vi "Sample changer.vi"() -> ()   [LabVIEW 2016, in "Top Level.lvlib"]
uses:
  Top Level.lvlib
  Sample Changer 2008 BETA 3.10.3/Visual Readback/half extended piston (push).ctl
  Sample Changer 2008 BETA 3.10.3/Visual Readback/half extended piston (push-in).ctl
  Sample Changer 2008 BETA 3.10.3/Visual Readback/Sample Rod (mid).ctl
  Sample Changer 2008 BETA 3.10.3/Visual Readback/Sample Rod (up-cathode).ctl
  Sample Changer 2008 BETA 3.10.3/Visual Readback/Sample Rod (down).ctl
  Sample Changer 2008 BETA 3.10.3/Visual Readback/Wheel Gate Valve.ctl
  cRIO code/SCA/controls/Horizontal Rod states.ctl
  cRIO code/SCA/controls/Vertical Rod states.ctl
  controls/GV states.ctl
  cRIO code/SCA/controls/SCA broadcast status.ctl
  cRIO code/SCA/controls/SCA Bypass control.ctl
  cRIO code/SCA/controls/GP307 cluster.ctl
  cRIO code/SCA/controls/SCA commands.ctl
panel:
  in  "Tab Control":T1(tab)=enum."SCA Configuration"
  out "Sample Rod (down)":T2
  in  "Random Change":bool
  in  "Random rotate":bool
  in  "Open SC GV":bool
  in  "Close SC GV":bool
  in  "Raise sample rod":bool
  in  "Lower sample rod":bool
  in  "Retract retract rod":bool
  in  "Insert retract rod":bool
  in  "pump out system":bool
  in  "Retract insert rod":bool
  in  "Insert insert rod":bool
  in  "Requested sample":i16=1 min=1 max=64 step=1
  in  "rotate wheel":bool
  in  "change sample":bool
  in  "vent system":bool
  out "Extended Piston (out)":bool
  out "half extended piston (out)":T3
  out "Extended Piston (in)":bool
  out "half extended piston (in)":T4
  out "Sample Rod (mid)":T5
  out "Sample Rod (up)":T6
  out "Wheel Gate Valve":T7
  in  "stop":bool
  out "SCA Status":T8
  out "Status Message":string
  out "Wheel GV Status":T9
  out "Insert Rod Status":T10
  out "Retract Rod Status":T10
  out "Sample Rod status":T11
  out "Bellows Pressure":string
  out "Source Pressure":string
  out "Encoder position":i16
  out "New sample":i8
  out "Encoder Destination":i16
  out "Encoder position plot":i16(graph)
  in  "Time between data points (ms)":u32=100
  out "Encoder Position":u32
  out "Encoder Offset":i16
  out "Insert Rod Timeout":u32
  out "Retract Rod Timeout":u32
  out "Rollover Sample":i16
  out "Wheel GV Timeout":u32
  out "Step Window Radius":u8
  out "Rotate Wheel min Time":u32
  out "Sample Rod Timeout":u32
  out "Rotate Wheel timeout":u32
  in  "SM Config Update?":bool
  in  "Bypass Controls":T12
  out "Bypass Control Values":T12
  in  "Encoder Offset set":i16
  in  "Insert Rod Timeout set":u32
  in  "Retract Rod Timeout set":u32
  in  "Step Window Radius set":u8
  in  "Rollover Sample set":i16
  in  "Rotate Wheel min Time set":u32
  in  "Rotate Wheel timeout set":u32
  in  "Sample Rod Timeout set":u32
  in  "Wheel GV Timeout set":u32
  out "Shared Network Variable Error":errorcluster
  out "Change sample error":errorcluster
  out "SCA-RT error":errorcluster
  out "Rotate Wheel error":errorcluster
  out "SM command error":errorcluster
  out "Random change error":errorcluster
  out "Random rotate error":errorcluster
  out "SM Config Update error":errorcluster
  # "Opens or Closes Wheel chamber valve"
  # "rotate wheel or change sample"
  # "Inserts sample into wheel"
  # "Pushes sample out of wheel"
  # "Raises or lowers Sample Rod"
  # "vent system= isolate wheel chamber from bellows and source\nPump out system = re-connect wheel chamber to bellows and source"
  # "In order for new settings to take effect must press Update? button.\nAll time values are in ms.  Encoder items are in encoder steps (0-2^14)"
  # "If the cathode position is too low: You have to increase the value. Too high, you have to lower it.\n\nEncoder radius is the minimum number of steps allowed between desired and actual position\n\nRollover sample is defined as the last sample before the standard encoder conversion exceeds 2^14"
  # "Current Values"
  # "New Values"
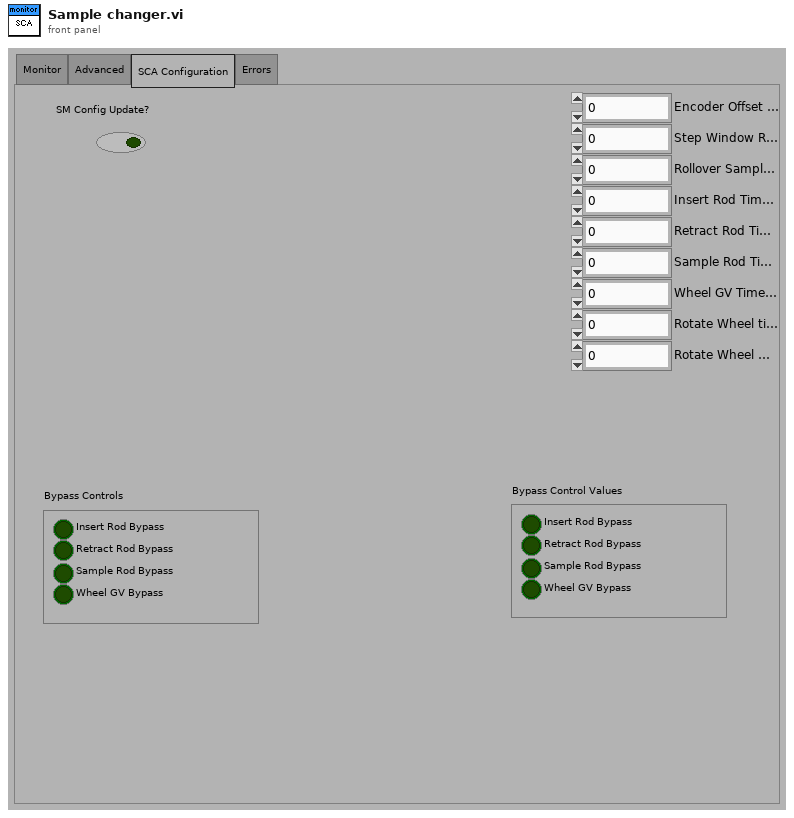
[diagram p1: front panel]
types:
  T1 = enum32{"Monitor", "Advanced", "SCA Configuration", "Errors"}
  T2 = typedef "Sample Rod (down).ctl" = bool
  T3 = typedef "half extended piston (push).ctl" = bool
  T4 = typedef "half extended piston (push-in).ctl" = bool
  T5 = typedef "Sample Rod (mid).ctl" = bool
  T6 = typedef "Sample Rod (up-cathode).ctl" = bool
  T7 = typedef "Wheel Gate Valve.ctl" = bool
  T8 = typedef "SCA broadcast status.ctl" = enum16{"Waiting", "Changing samples", "Sample change complete", "Failure"}
  T9 = typedef "GV states.ctl" = enum16{"status unclear", "closed", "open"}
  T10 = typedef "Horizontal Rod states.ctl" = enum16{"status unclear", "rod in", "rod out"}
  T11 = typedef "Vertical Rod states.ctl" = enum16{"status unclear", "rod down", "rod up"}
  T12 = typedef "SCA Bypass control.ctl" = cluster{"Insert Rod Bypass":bool, "Retract Rod Bypass":bool, "Sample Rod Bypass":bool, "Wheel GV Bypass":bool}
  T13 = typedef "SCA commands.ctl" = enum16{"Wait", "Shutdown", "Retract insert rod", "Insert insert rod", "Retract retract rod", "Insert retract rod", "Retract sample rod", "Insert sample rod", "Open wheel GV", "Close wheel GV", "Open ion source GV", "Close ion source GV", "Pump out source", "Vent source", "Rotate wheel randomly", "Rotate wheel", "Start random sample change", "Start sample change"}
  T14 = typedef "GP307 cluster.ctl" = cluster{"Ion gauge 1":string, "Convectron  Gauge 1 ":string, "Ion Gauge 2":string, "Convectrom Gauge 2":string}
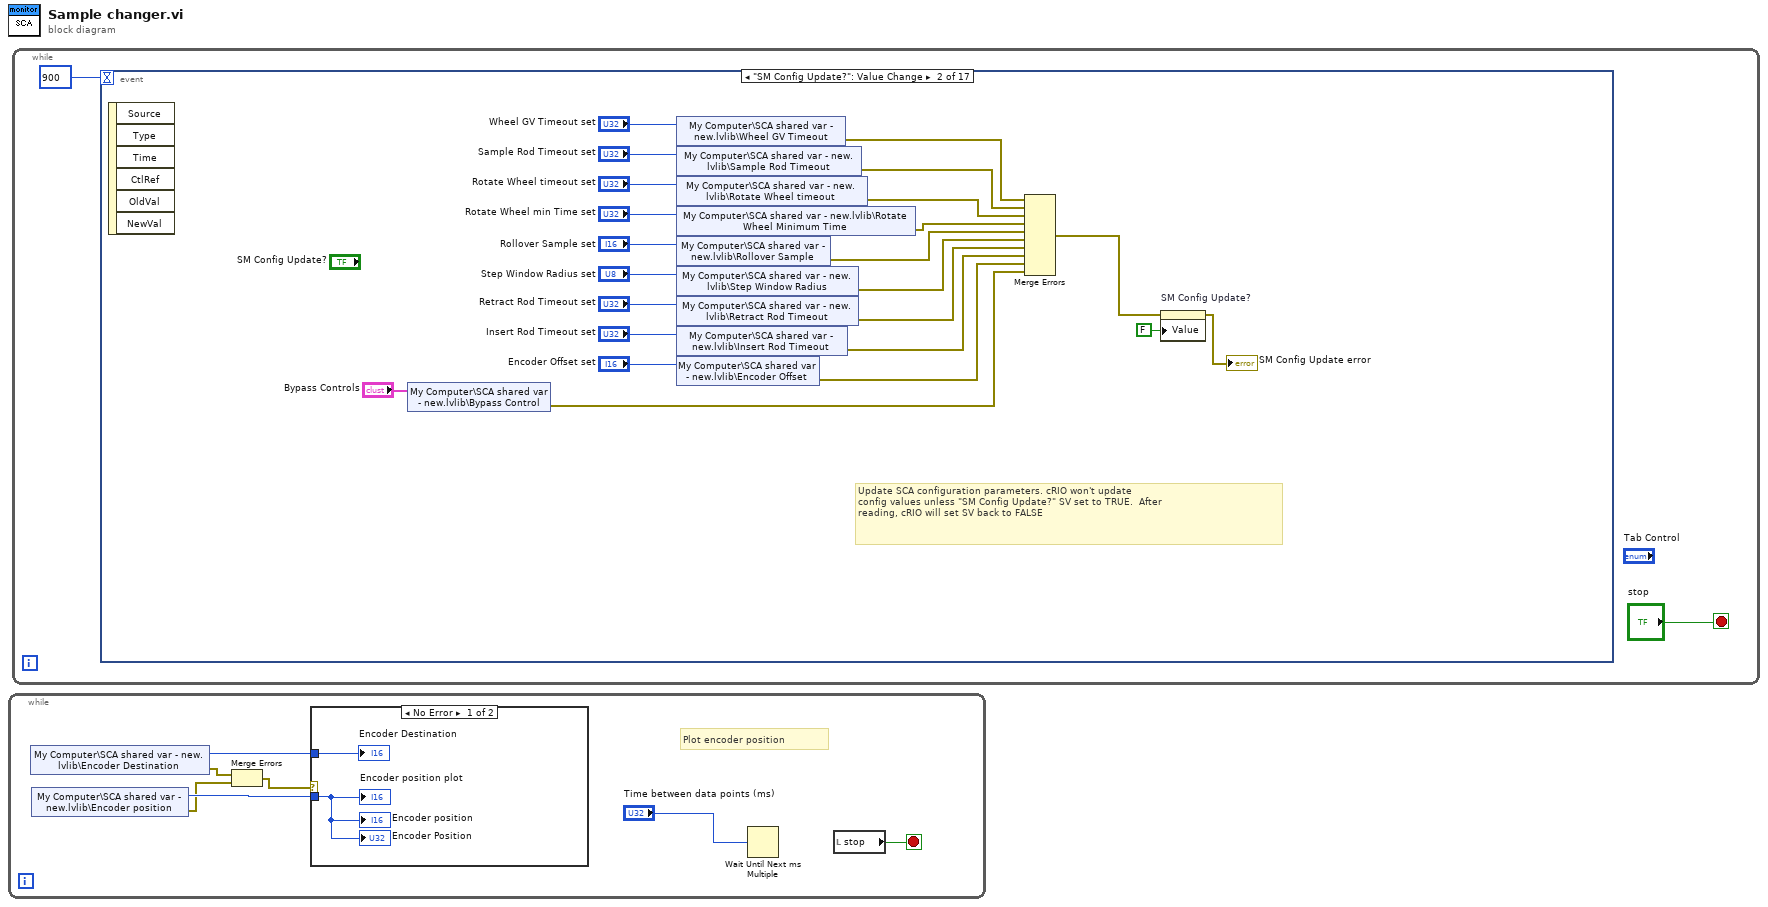
[diagram p0: block diagram]
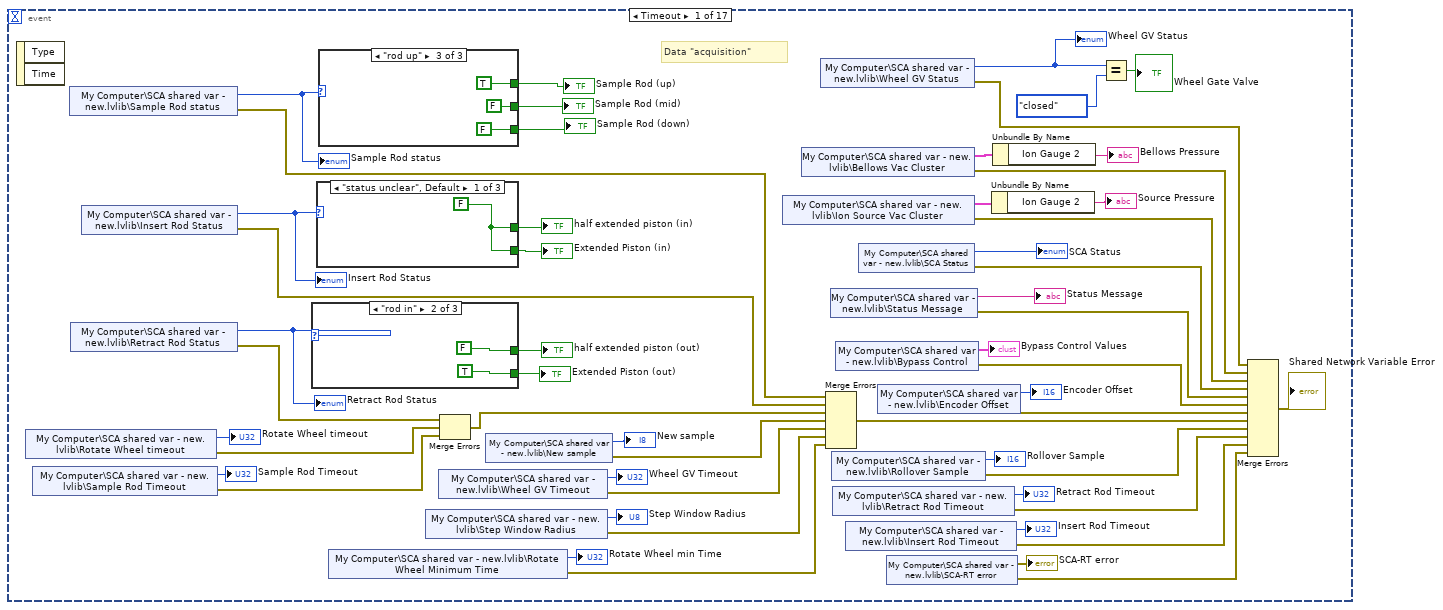
[diagram p3: hidden frame]
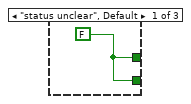
[diagram p4: hidden frame]
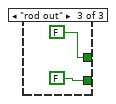
[diagram p5: hidden frame]
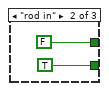
[diagram p6: hidden frame]
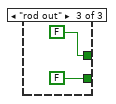
[diagram p7: hidden frame]
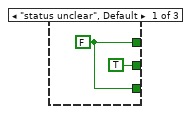
[diagram p8: hidden frame]
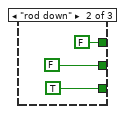
[diagram p9: hidden frame]
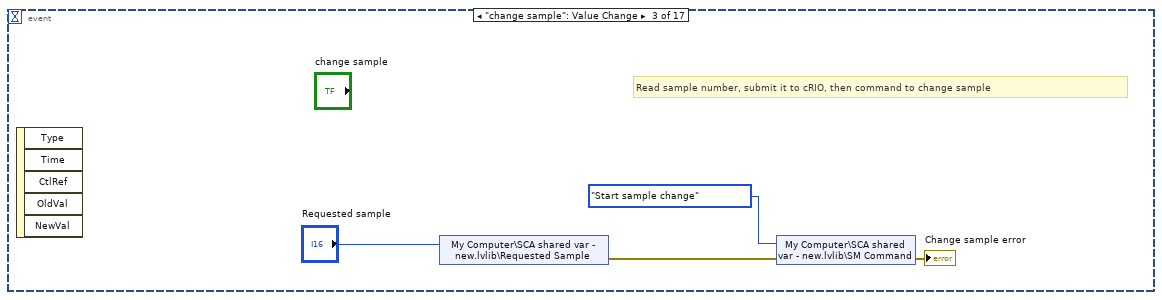
[diagram p10: hidden frame]
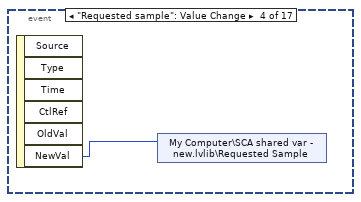
[diagram p11: hidden frame]
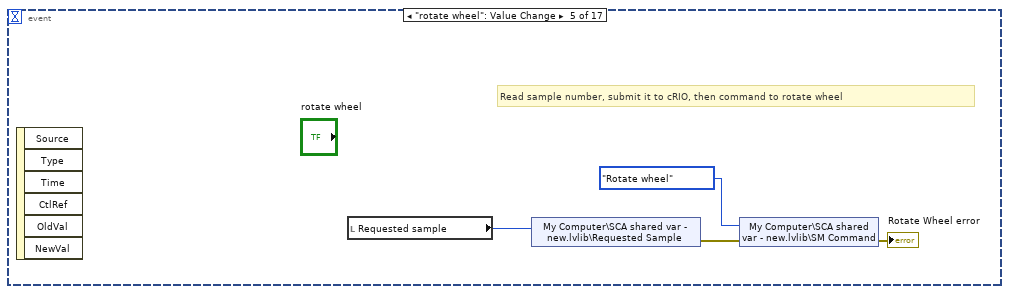
[diagram p12: hidden frame]
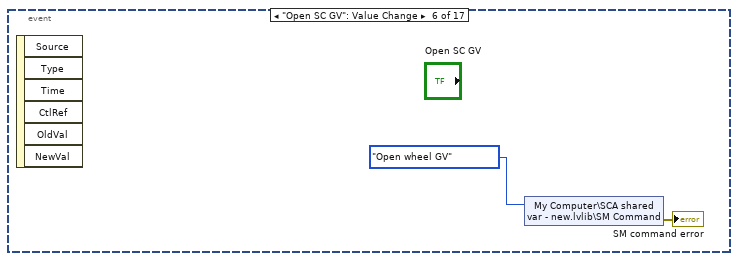
[diagram p13: hidden frame]
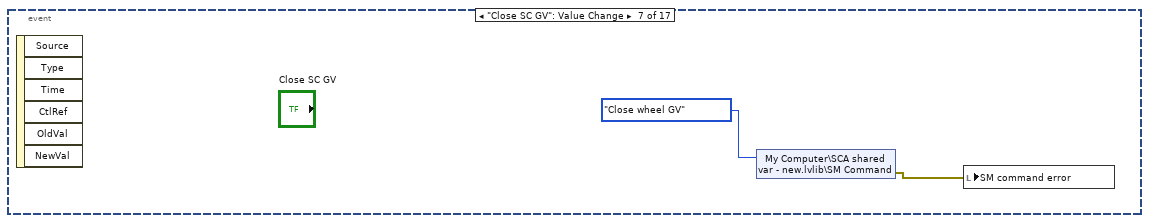
[diagram p14: hidden frame]
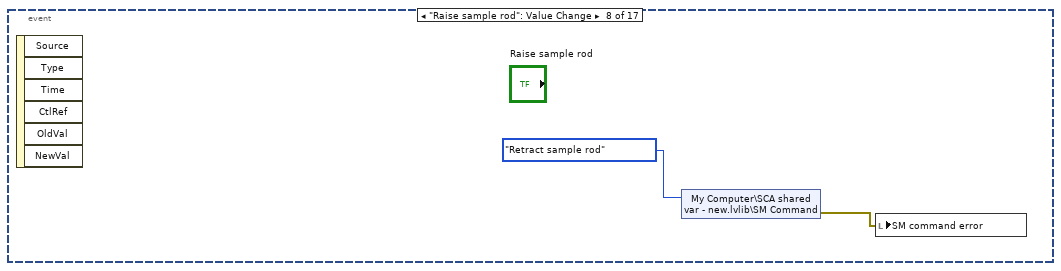
[diagram p15: hidden frame]
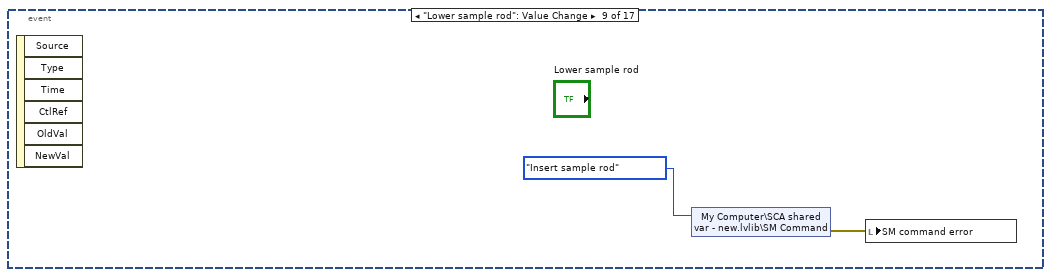
[diagram p16: hidden frame]
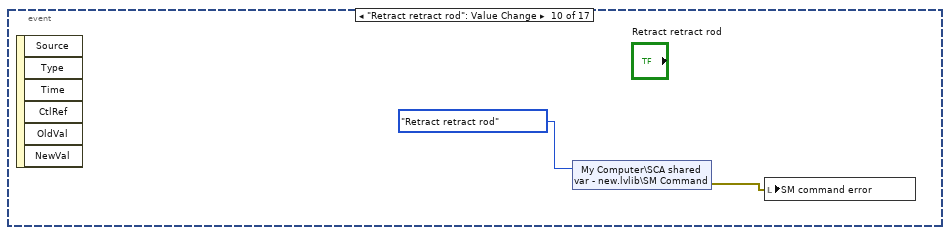
[diagram p17: hidden frame]
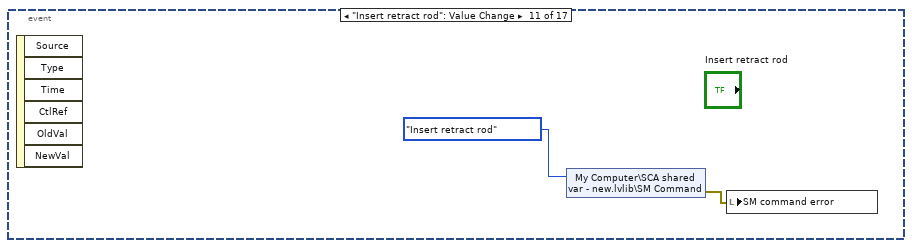
[diagram p18: hidden frame]
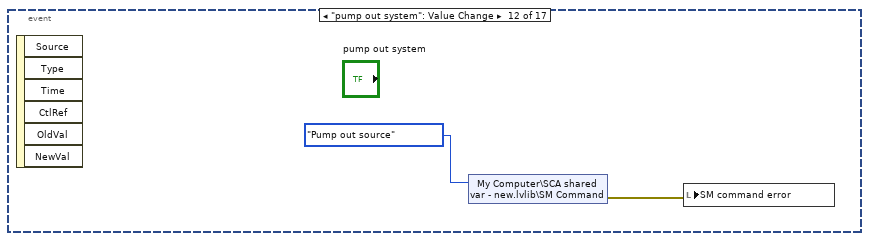
[diagram p19: hidden frame]
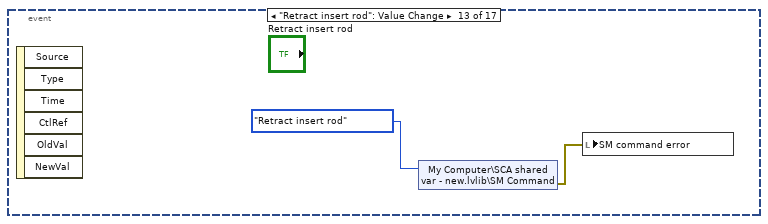
[diagram p20: hidden frame]
diagram:
  n1 = while {
    stop <- w4 stop-if-true
    # "Plot encoder position"
    n2 = shared-variable "My Computer\\SCA shared var - new.lvlib\\Encoder Destination"() -> (w7:i16, error out=w3:errorcluster)  [unwired: 1 in]
    n3 = shared-variable "My Computer\\SCA shared var - new.lvlib\\Encoder position"() -> (w5:i16, error out=w2:errorcluster)  [unwired: 1 in]
    n4 = Merge Errors(w3, w2) -> (w1:errorcluster)
    n5 = case shown="No Error" w1 {
      tunnel: w7 -> [w9 _]
      tunnel: w5 -> [w8 _]
      frame No Error {
        "Encoder Destination" <- w9
        "Encoder position plot" <- w8
        "Encoder Position" <- w8
        "Encoder position" <- w8
      }
      frame Error {
      }
    }
    n6 = Wait Until Next ms Multiple(millisecond multiple="Time between data points (ms)") -> ()  [unwired: 1 out]
    n7 = local read "stop"() -> (w4:bool)
  }
  n8 = while {
    stop <- "stop" stop-if-true
    n9 = event shown="[1] \"SM Config Update?\": Value Change" {
      selector: _ -> [_ _ _ _ _ _ _ _ _ _ _ _ _ _ _ _ _]
      dyn-events: _ -> [_ _ _ _ _ _ _ _ _ _ _ _ _ _ _ _ _]
      timeout: 900 -> [_ _ _ _ _ _ _ _ _ _ _ _ _ _ _ _ _]
      event Timeout {
        # "Data \"acquisition\""
        n10 = event-data() -> ()  [unwired: 1 in, 2 out]
        n11 = shared-variable "My Computer\\SCA shared var - new.lvlib\\Rotate Wheel timeout"() -> (→"Rotate Wheel timeout":u32, error out=w13:errorcluster)  [unwired: 1 in]
        n12 = shared-variable "My Computer\\SCA shared var - new.lvlib\\Sample Rod Timeout"() -> (→"Sample Rod Timeout":u32, error out=w12:errorcluster)  [unwired: 1 in]
        n13 = shared-variable "My Computer\\SCA shared var - new.lvlib\\Sample Rod status"() -> (w65:T11, error out=w38:errorcluster)  [unwired: 1 in]
        "Sample Rod status" <- w65
        n14 = shared-variable "My Computer\\SCA shared var - new.lvlib\\Retract Rod Status"() -> (w59:T10, error out=w36:errorcluster)  [unwired: 1 in]
        "Retract Rod Status" <- w59
        n15 = shared-variable "My Computer\\SCA shared var - new.lvlib\\Insert Rod Status"() -> (w56:T10, error out=w37:errorcluster)  [unwired: 1 in]
        "Insert Rod Status" <- w56
        n16 = case shown="\"rod in\"" w59 {
          tunnel: [w66 TRUE FALSE] -> w60
          tunnel: [w66 FALSE FALSE ("Time Out Occured")] -> w61
          frame "status unclear", Default {
            w66 = FALSE ("Time Out Occured")
          }
          frame "rod in" {
          }
          frame "rod out" {
          }
        }
        "Extended Piston (out)" <- w60
        "half extended piston (out)" <- w61
        n17 = case shown="\"status unclear\", Default" w56 {
          tunnel: [w71 TRUE FALSE] -> w58
          tunnel: [w71 FALSE FALSE ("Time Out Occured")] -> w57
          frame "status unclear", Default {
            w71 = FALSE ("Time Out Occured")
          }
          frame "rod in" {
          }
          frame "rod out" {
          }
        }
        "Extended Piston (in)" <- w58
        "half extended piston (in)" <- w57
        n18 = case shown="\"rod up\"" w65 {
          tunnel: [w77 TRUE FALSE] -> w62
          tunnel: [TRUE ("Time Out Occured") FALSE FALSE ("Time Out Occured")] -> w63
          tunnel: [w77 FALSE ("Time Out Occured") TRUE ("Time Out Occured")] -> w64
          frame "status unclear", Default {
            w77 = FALSE ("Time Out Occured")
          }
          frame "rod down" {
          }
          frame "rod up" {
          }
        }
        "Sample Rod (mid)" <- w63
        "Sample Rod (up)" <- w64
        "Sample Rod (down)" <- w62
        n19 = shared-variable "My Computer\\SCA shared var - new.lvlib\\Rotate Wheel Minimum Time"() -> (→"Rotate Wheel min Time":u32, error out=w17:errorcluster)  [unwired: 1 in]
        n20 = shared-variable "My Computer\\SCA shared var - new.lvlib\\Step Window Radius"() -> (→"Step Window Radius":u8, error out=w18:errorcluster)  [unwired: 1 in]
        n21 = shared-variable "My Computer\\SCA shared var - new.lvlib\\Wheel GV Timeout"() -> (→"Wheel GV Timeout":u32, error out=w19:errorcluster)  [unwired: 1 in]
        n22 = Merge Errors(w36, w13, w12) -> (w14:errorcluster)
        n23 = shared-variable "My Computer\\SCA shared var - new.lvlib\\New sample"() -> (→"New sample":i8, error out=w31:errorcluster)  [unwired: 1 in]
        n24 = shared-variable "My Computer\\SCA shared var - new.lvlib\\Ion Source Vac Cluster"() -> (w54:T14, error out=w46:errorcluster)  [unwired: 1 in]
        n25 = shared-variable "My Computer\\SCA shared var - new.lvlib\\Bellows Vac Cluster"() -> (w55:T14, error out=w47:errorcluster)  [unwired: 1 in]
        n26 = shared-variable "My Computer\\SCA shared var - new.lvlib\\Wheel GV Status"() -> (w51:T9, error out=w48:errorcluster)  [unwired: 1 in]
        "Wheel GV Status" <- w51
        n27 = Merge Errors(w38, w37, w14, w31, w19, w18, w17) -> (w35:errorcluster)
        n28 = shared-variable "My Computer\\SCA shared var - new.lvlib\\Status Message"() -> (→"Status Message":string, error out=w41:errorcluster)  [unwired: 1 in]
        n29 = shared-variable "My Computer\\SCA shared var - new.lvlib\\Rollover Sample"() -> (→"Rollover Sample":i16, error out=w23:errorcluster)  [unwired: 1 in]
        n30 = shared-variable "My Computer\\SCA shared var - new.lvlib\\Retract Rod Timeout"() -> (→"Retract Rod Timeout":u32, error out=w27:errorcluster)  [unwired: 1 in]
        n31 = shared-variable "My Computer\\SCA shared var - new.lvlib\\Bypass Control"() -> (→"Bypass Control Values":T12, error out=w40:errorcluster)  [unwired: 1 in]
        n32 = shared-variable "My Computer\\SCA shared var - new.lvlib\\Insert Rod Timeout"() -> (→"Insert Rod Timeout":u32, error out=w28:errorcluster)  [unwired: 1 in]
        n33 = shared-variable "My Computer\\SCA shared var - new.lvlib\\SCA Status"() -> (→"SCA Status":T8, error out=w42:errorcluster)  [unwired: 1 in]
        n34 = shared-variable "My Computer\\SCA shared var - new.lvlib\\Encoder Offset"() -> (→"Encoder Offset":i16, error out=w30:errorcluster)  [unwired: 1 in]
        n35 = shared-variable "My Computer\\SCA shared var - new.lvlib\\SCA-RT error"() -> (→"SCA-RT error":errorcluster, error out=w33:errorcluster)  [unwired: 1 in]
        n36 = Unbundle By Name(w54) -> ("Ion Gauge 2"=→"Source Pressure":string)
        n37 = Unbundle By Name(w55) -> ("Ion Gauge 2"=→"Bellows Pressure":string)
        n38 = Equal?(x=w51, y=GV_states."closed") -> (x = y?=→"Wheel Gate Valve":bool)
        n39 = Merge Errors(w48, w47, w46, w42, w41, w40, w30, w35, w23, w27, w28, w33) -> (→"Shared Network Variable Error":errorcluster)
      }
      event "SM Config Update?": Value Change {
        # "Update SCA configuration parameters. cRIO won't update\nconfig values unless \"SM Config Update?\" SV set to TRUE.  After\nreading, cRIO will set SV back to FALSE"
        n40 = event-data() -> ()  [unwired: 1 in, 6 out]
        n41 = shared-variable "My Computer\\SCA shared var - new.lvlib\\Bypass Control"("Bypass Controls") -> (error out=w86:errorcluster)  [unwired: 1 in]
        n42 = shared-variable "My Computer\\SCA shared var - new.lvlib\\Wheel GV Timeout"("Wheel GV Timeout set") -> (error out=w95:errorcluster)  [unwired: 1 in]
        n43 = shared-variable "My Computer\\SCA shared var - new.lvlib\\Sample Rod Timeout"("Sample Rod Timeout set") -> (error out=w94:errorcluster)  [unwired: 1 in]
        n44 = shared-variable "My Computer\\SCA shared var - new.lvlib\\Rotate Wheel timeout"("Rotate Wheel timeout set") -> (error out=w93:errorcluster)  [unwired: 1 in]
        n45 = shared-variable "My Computer\\SCA shared var - new.lvlib\\Rotate Wheel Minimum Time"("Rotate Wheel min Time set") -> (error out=w92:errorcluster)  [unwired: 1 in]
        n46 = shared-variable "My Computer\\SCA shared var - new.lvlib\\Rollover Sample"("Rollover Sample set") -> (error out=w91:errorcluster)  [unwired: 1 in]
        n47 = shared-variable "My Computer\\SCA shared var - new.lvlib\\Step Window Radius"("Step Window Radius set") -> (error out=w90:errorcluster)  [unwired: 1 in]
        n48 = shared-variable "My Computer\\SCA shared var - new.lvlib\\Retract Rod Timeout"("Retract Rod Timeout set") -> (error out=w89:errorcluster)  [unwired: 1 in]
        n49 = shared-variable "My Computer\\SCA shared var - new.lvlib\\Insert Rod Timeout"("Insert Rod Timeout set") -> (error out=w88:errorcluster)  [unwired: 1 in]
        n50 = shared-variable "My Computer\\SCA shared var - new.lvlib\\Encoder Offset"("Encoder Offset set") -> (error out=w87:errorcluster)  [unwired: 1 in]
        n51 = Merge Errors(w95, w94, w93, w92, w91, w90, w89, w88, w87, w86) -> (w85:errorcluster)
        n52 = property on="SM Config Update?" class="Bool (strict)"(error in=w85, "Value"=FALSE ("SM Config Update?")) -> (error out=→"SM Config Update error":errorcluster)  [unwired: 1 in, 1 out]
      }
      event "change sample": Value Change {
        # "Read sample number, submit it to cRIO, then command to change sample"
        n53 = event-data() -> ()  [unwired: 1 in, 5 out]
        n54 = shared-variable "My Computer\\SCA shared var - new.lvlib\\Requested Sample"("Requested sample") -> (error out=w107:errorcluster)  [unwired: 1 in]
        n55 = shared-variable "My Computer\\SCA shared var - new.lvlib\\SM Command"(SCA_commands."Start sample change" ("SM Command"), error in=w107) -> (error out=→"Change sample error":errorcluster)
      }
      event "Requested sample": Value Change {
        n56 = event-data() -> ("NewVal"=w111:i16)  [unwired: 1 in, 5 out]
        n57 = shared-variable "My Computer\\SCA shared var - new.lvlib\\Requested Sample"(w111) -> ()  [unwired: 1 in, 1 out]
      }
      event "rotate wheel": Value Change {
        # "Read sample number, submit it to cRIO, then command to rotate wheel"
        n58 = event-data() -> ()  [unwired: 1 in, 6 out]
        n59 = local read "Requested sample"() -> (w115:i16)
        n60 = shared-variable "My Computer\\SCA shared var - new.lvlib\\Requested Sample"(w115) -> (error out=w114:errorcluster)  [unwired: 1 in]
        n61 = shared-variable "My Computer\\SCA shared var - new.lvlib\\SM Command"(SCA_commands."Rotate wheel" ("SM Command"), error in=w114) -> (error out=→"Rotate Wheel error":errorcluster)
      }
      event "Open SC GV": Value Change {
        n62 = event-data() -> ()  [unwired: 1 in, 6 out]
        n63 = shared-variable "My Computer\\SCA shared var - new.lvlib\\SM Command"(SCA_commands."Open wheel GV" ("SM Command")) -> (error out=→"SM command error":errorcluster)  [unwired: 1 in]
      }
      event "Close SC GV": Value Change {
        n64 = event-data() -> ()  [unwired: 1 in, 6 out]
        n65 = shared-variable "My Computer\\SCA shared var - new.lvlib\\SM Command"(SCA_commands."Close wheel GV" ("SM Command")) -> (error out=w118:errorcluster)  [unwired: 1 in]
        n66 = local write "SM command error"(w118) -> ()
      }
      event "Raise sample rod": Value Change {
        n67 = event-data() -> ()  [unwired: 1 in, 6 out]
        n68 = shared-variable "My Computer\\SCA shared var - new.lvlib\\SM Command"(SCA_commands."Retract sample rod" ("SM Command")) -> (error out=w120:errorcluster)  [unwired: 1 in]
        n69 = local write "SM command error"(w120) -> ()
      }
      event "Lower sample rod": Value Change {
        n70 = event-data() -> ()  [unwired: 1 in, 6 out]
        n71 = shared-variable "My Computer\\SCA shared var - new.lvlib\\SM Command"(SCA_commands."Insert sample rod" ("SM Command")) -> (error out=w122:errorcluster)  [unwired: 1 in]
        n72 = local write "SM command error"(w122) -> ()
      }
      event "Retract retract rod": Value Change {
        n73 = event-data() -> ()  [unwired: 1 in, 6 out]
        n74 = shared-variable "My Computer\\SCA shared var - new.lvlib\\SM Command"(SCA_commands."Retract retract rod" ("SM Command")) -> (error out=w124:errorcluster)  [unwired: 1 in]
        n75 = local write "SM command error"(w124) -> ()
      }
      event "Insert retract rod": Value Change {
        n76 = event-data() -> ()  [unwired: 1 in, 6 out]
        n77 = shared-variable "My Computer\\SCA shared var - new.lvlib\\SM Command"(SCA_commands."Insert retract rod" ("SM Command")) -> (error out=w126:errorcluster)  [unwired: 1 in]
        n78 = local write "SM command error"(w126) -> ()
      }
      event "pump out system": Value Change {
        n79 = event-data() -> ()  [unwired: 1 in, 6 out]
        n80 = shared-variable "My Computer\\SCA shared var - new.lvlib\\SM Command"(SCA_commands."Pump out source" ("SM Command")) -> (error out=w128:errorcluster)  [unwired: 1 in]
        n81 = local write "SM command error"(w128) -> ()
      }
      event "Retract insert rod": Value Change {
        n82 = event-data() -> ()  [unwired: 1 in, 6 out]
        n83 = shared-variable "My Computer\\SCA shared var - new.lvlib\\SM Command"(SCA_commands."Retract insert rod" ("SM Command")) -> (error out=w130:errorcluster)  [unwired: 1 in]
        n84 = local write "SM command error"(w130) -> ()
      }
      event "Insert insert rod": Value Change {
        n85 = event-data() -> ()  [unwired: 1 in, 6 out]
        n86 = shared-variable "My Computer\\SCA shared var - new.lvlib\\SM Command"(SCA_commands."Insert insert rod" ("SM Command")) -> (error out=w132:errorcluster)  [unwired: 1 in]
        n87 = local write "SM command error"(w132) -> ()
      }
      event "vent system": Value Change {
        n88 = event-data() -> ()  [unwired: 1 in, 6 out]
        n89 = shared-variable "My Computer\\SCA shared var - new.lvlib\\SM Command"(SCA_commands."Vent source" ("SM Command")) -> (error out=w134:errorcluster)  [unwired: 1 in]
        n90 = local write "SM command error"(w134) -> ()
      }
      event "Random rotate": Value Change {
        n91 = event-data() -> ()  [unwired: 1 in, 6 out]
        n92 = shared-variable "My Computer\\SCA shared var - new.lvlib\\SM Command"(SCA_commands."Rotate wheel randomly" ("SM Command")) -> (error out=→"Random rotate error":errorcluster)  [unwired: 1 in]
      }
      event "Random Change": Value Change {
        n93 = event-data() -> ()  [unwired: 1 in, 6 out]
        n94 = shared-variable "My Computer\\SCA shared var - new.lvlib\\SM Command"(SCA_commands."Start random sample change" ("SM Command")) -> (error out=→"Random change error":errorcluster)  [unwired: 1 in]
      }
    }
  }
